vi "FromRepo.vi"(8 "error in":errorcluster, 9 "from repo cluster":T2, 10 "repository in":refnum<class "NISE_CEF_Repository.lvclass">, 11 "node in":refnum<class "CustomDevice.lvclass">) -> (0 "error out":errorcluster, 2 "repository out":refnum<class "NISE_CEF_Repository.lvclass">, 3 "node":T1)   [LabVIEW 2015, in "CustomDevice.lvclass"]
doc: "Grabs information from the Repo and stores it in the nodes."
uses:
  CustomDevice.lvclass
  <vilib>/NI/Configuration Framework/Repository/NISE_CEF_Repository.lvclass
  <vilib>/NI/Configuration Framework/Node/FromRepoCluster.ctl
  <vilib>/NI/Configuration Framework/Node/NodeRef.ctl
  <vilib>/NI/Configuration Framework/Node/NISE_CEF_Node.lvclass
  CustomDeviceRepo/CustomDeviceRepo.lvclass
  CustomDeviceRepo/CustomDeviceRepo.lvclass/CustomDeviceRepo.ctl
  CustomDevice.lvclass/CustomDevice.ctl
  CustomDeviceRepo/Read Main CD Properties.vi
  CustomDeviceRepo/Read Timing Source Properties.vi
  Write Main CD Properties.vi
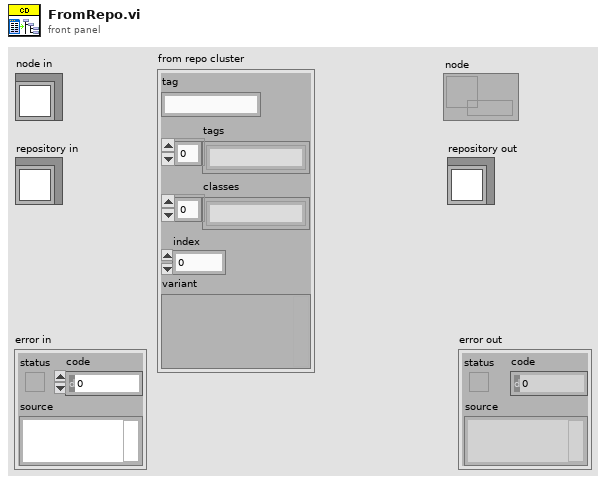
[diagram p1: front panel]
types:
  T1 = typedef "NISE_CEF_Node.lvclass/NodeRef.ctl" = refnum<data-value>
  T2 = typedef "NISE_CEF_Node.lvclass/FromRepoCluster.ctl" = cluster{"tag":string, "tags":string[], "classes":string[], "index":i32, "variant":variant}
  T3 = typedef "Main Custom Device Properties.ctl" = cluster{"CD Name":string, "Version":string, "Max Occurrences":i32, "Device Type":enum16{"Asynchronous", "Inline HW Interface", "Inline Model Interface", "Inline Timing and Sync", "Asynchronous Timing and Sync"}, "Main Page GUID":string}
  T4 = typedef "Timing Source Properties.ctl" = cluster{"Has Timing Source Capability":bool, "Source Distribution":T5}
  T5 = typedef "Source Distribution for TimingSource.ctl" = cluster{"Supported Target":T6, "Source":T7, "Real Time System Destination":string, "Version":string}[]
  T6 = typedef "Target.ctl" = enum16{"All", "Pharlap", "VxWorks", "Windows", "Linux_32_ARM", "Linux_x64", "PharlapWindows", "PharlapVxWorks", "VxWorksWindows"}
  T7 = typedef "Path Cluster.ctl" = cluster{"Path":path, "Path Type":enum16{"Absolute", "To Base", "To Common Doc Dir", "To Application Data Dir"}}
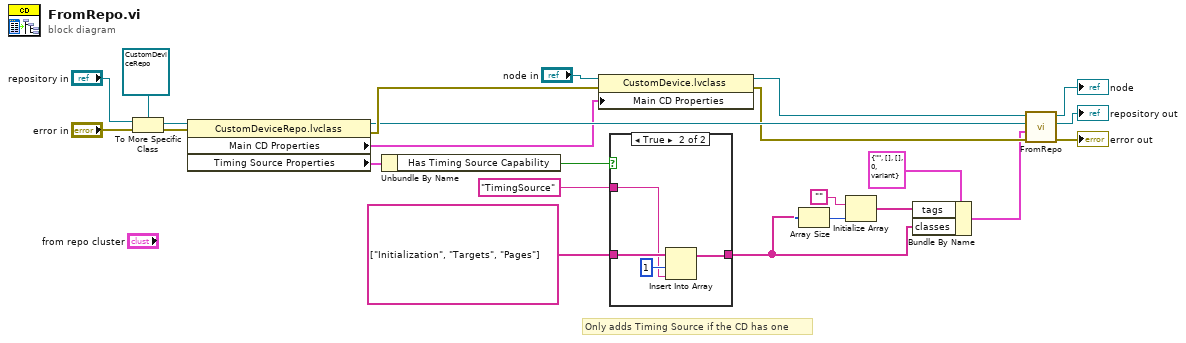
[diagram p0: block diagram]
diagram:
  # "Only adds Timing Source if the CD has one"
  n1 = To More Specific Class(target class=refnum<class "CustomDeviceRepo.lvclass"> refnum ("CustomDeviceRepo.lvclass"), reference="repository in", error in="error in") -> (specific class reference=w18:refnum<class "CustomDeviceRepo.lvclass">, error out=w17:errorcluster)
  n2 = property class="CustomDeviceRepo.lvclass"(reference=w18, error in=w17) -> (reference out=w13:refnum<class "CustomDeviceRepo.lvclass">, error out=w15:errorcluster, "Main CD Properties"=w11:T3, "Timing Source Properties"=w5:T4)
  n3 = Unbundle By Name(w5) -> ("Has Timing Source Capability"=w4:bool)
  n4 = property class="CustomDevice.lvclass"(reference="node in", error in=w15, "Main CD Properties"=w11) -> (reference out=w14:refnum<class "CustomDevice.lvclass">, error out=w12:errorcluster)
  n5 = case shown="True" w4 {
    tunnel: string[] ["Initialization", "Targets", "Pages"] -> [w25 w29]
    tunnel: [w25 w26] -> w2
    tunnel: "TimingSource" -> [_ w27]
    frame False {
    }
    frame True {
      n6 = Insert Into Array(array=w29, index=1, new element=w27) -> (w26:string[])
    }
  }
  n7 = Array Size(array=w2) -> (size(s)=w6:i32)
  n8 = Initialize Array("", w6) -> (w7:string[])
  n9 = Bundle By Name(cluster=T2 {"tag"="", "tags"=[], "classes"=[], "index"=0, "variant"=variant} ("from repo cluster"), "tags"=w7, "classes"=w2) -> (w9:T2)
  n10 = call-parent "FromRepo.vi"("error in"=w12, "from repo cluster"=w9, "repository in"=w13, "node in"=w14) -> ("error out"=→"error out":errorcluster, "repository out"=→"repository out":refnum<class "NISE_CEF_Repository.lvclass">, "node"=→"node":T1)  [unwired: 5 in]
